vi "Read_CommandOrigin.vi"(8 "error in (no error)":errorcluster, 11 "SubsystemData in":refnum<class "SubsystemData.lvclass">) -> (0 "error out":errorcluster, 2 "Command Origin":T1, 3 "SubsystemData out":refnum<class "SubsystemData.lvclass">)   [LabVIEW 2017, in "SubsystemData.lvclass"]
uses:
  SubsystemData.lvclass
  CommandOrigin.ctl
  SubsystemData.lvclass/SubsystemData.ctl
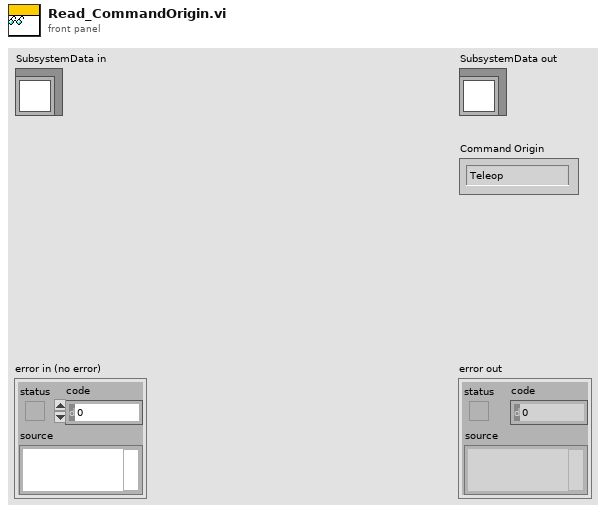
[diagram p1: front panel]
types:
  T1 = typedef "SubsystemData.lvclass/CommandOrigin.ctl" = enum16{"Teleop", "Auto"}
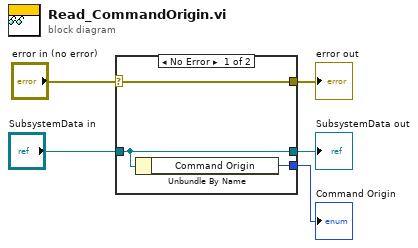
[diagram p0: block diagram]
diagram:
  n1 = case shown="No Error" "error in (no error)" {
    selector: "error in (no error)" -> [w8 w9]
    tunnel: [w8 w9] -> w4
    tunnel: [w7 w10] -> w2
    tunnel: "SubsystemData in" -> [w7 w10]
    tunnel: [w6 _] -> w1
    frame No Error {
      n2 = Unbundle By Name(w7) -> ("Command Origin"=w6:T1)
    }
    frame Error {
    }
  }
  "error out" <- w4
  "SubsystemData out" <- w2
  "Command Origin" <- w1
